vi "Retreive Target BuildSpecs.vi"(8 "error in (no error)":errorcluster, 10 "Target Names in":string[](array[string]), 11 "Project Sync Tools in":refnum<class "Project Sync Tools.lvclass">) -> (0 "error out":errorcluster, 2 "Target Names out":string[](array[string]), 3 "Project Sync Tools out":refnum<class "Project Sync Tools.lvclass">)   [LabVIEW 2019, in "Project Sync Tools.lvclass"]
uses:
  Project Sync Tools.lvclass
  TypeDefs/BuildSpec Parameters.ctl
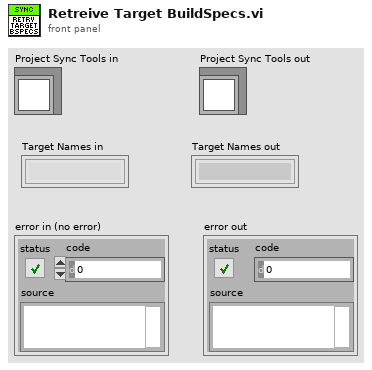
[diagram p1: front panel]
types:
  T1 = typedef "Project Sync Tools.lvclass/BuildSpec Parameters.ctl" = cluster{"BuildSpec Ref":refnum<vi>, "Target Name":string, "Build Spec Name":string, "Tags":string[], "Tag Values":variant[]}
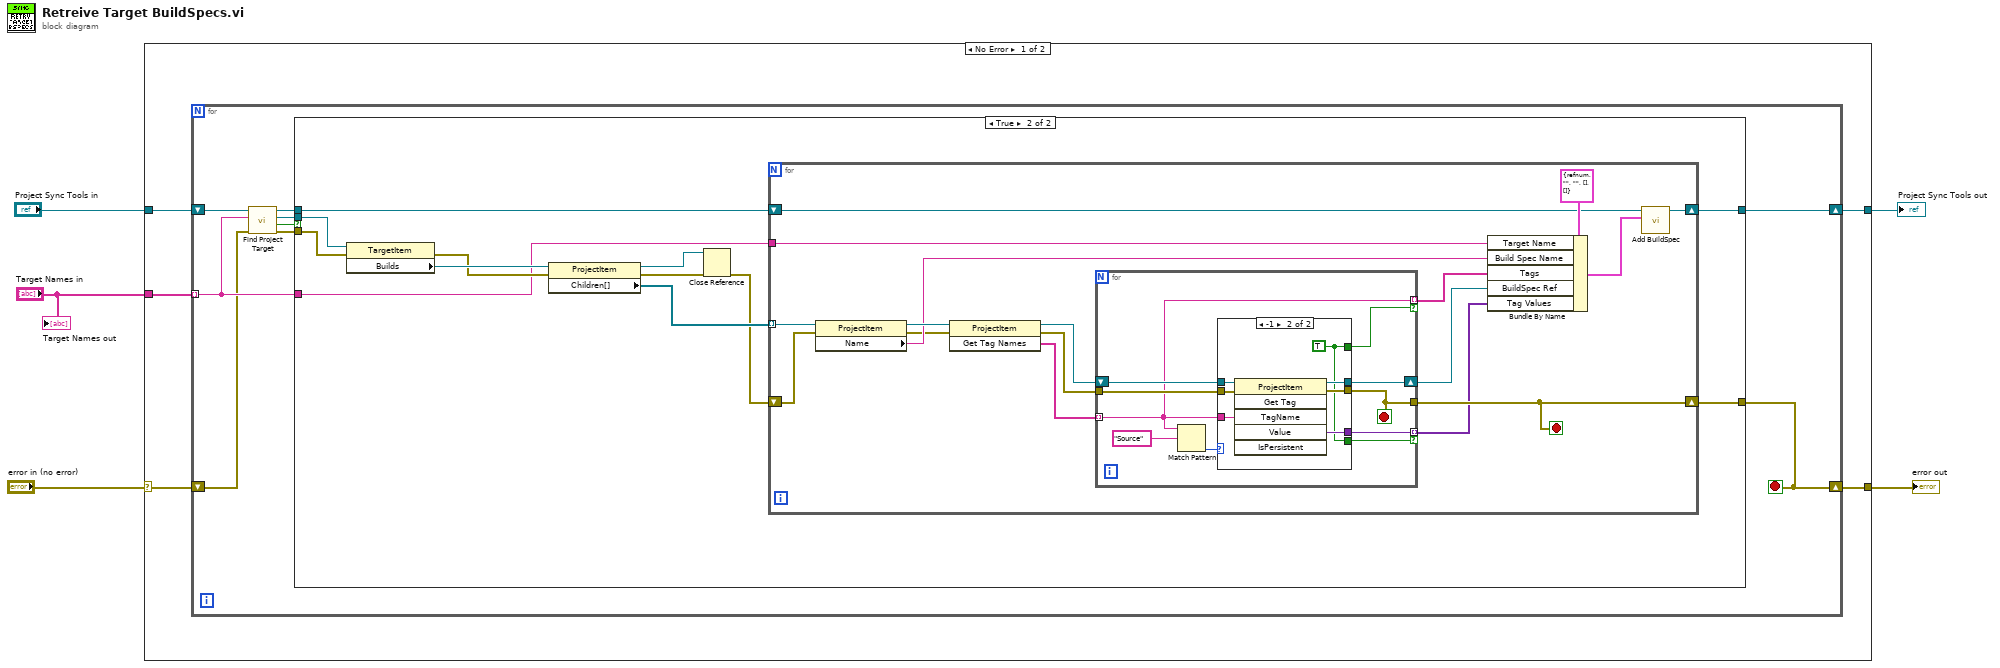
[diagram p0: block diagram]
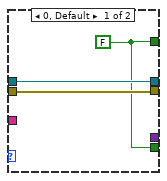
[diagram p3: hidden frame]
diagram:
  n1 = case shown="No Error" "error in (no error)" {
    selector: "error in (no error)" -> [w6 w72]
    tunnel: [w10 w71] -> w5
    tunnel: "Project Sync Tools in" -> [w9 w71]
    tunnel: "Target Names in" -> [w8 _]
    tunnel: [w7 w72] -> w3
    frame No Error {
      n2 = for {
        tunnel: w8 -> [w13] mode=indexing
        shift-right: [w19] -> w10
        shift-left: w9 -> [w17]
        shift-right: [w18] -> w7
        shift-left: w6 -> [w12]
        stop <- w18 stop-if-true
        n3 = call "Find Project Target.vi"("error in (no error)"=w12, "Target Name"=w13, "Project Sync Tools in"=w17) -> ("error out"=w11:errorcluster, "Found ?"=w16:bool, "TargetItem out"=w15:refnum<vi>, "Project Sync Tools out"=w14:refnum<class "Project Sync Tools.lvclass">)  [unwired: 5 in]
        n4 = case shown="True" w16 {
          tunnel: [w21 w31] -> w19
          tunnel: [w20 w27] -> w18
          tunnel: w15 -> [_ w25]
          tunnel: w14 -> [w21 w26]
          tunnel: w13 -> [_ w22]
          tunnel: w11 -> [w20 w24]
          frame False {
          }
          frame True {
            n5 = property class="TargetItem"(reference=w25, error in=w24) -> (error out=w23:errorcluster, "Builds"=w33:refnum<vi>)  [unwired: 1 out]
            n6 = property class="ProjectItem"(reference=w33, error in=w23) -> (reference out=w29:refnum<vi>, error out=w30:errorcluster, "Children[]"=w32:refnum<vi>[])
            n7 = Close Reference(reference=w29, error in (no error)=w30) -> (error out=w28:errorcluster)
            n8 = for {
              tunnel: w32 -> [w44] mode=indexing
              shift-right: [w45] -> w31
              shift-left: w26 -> [w46]
              tunnel: w22 -> [w42]
              shift-right: [w37] -> w27
              shift-left: w28 -> [w41]
              stop <- w37 stop-if-true
              n9 = property class="ProjectItem"(reference=w44, error in=w41) -> (reference out=w43:refnum<vi>, error out=w39:errorcluster, "Name"=w40:string)
              n10 = invoke class="ProjectItem" method="Get Tag Names"(reference=w43, error in=w39) -> (reference out=w50:refnum<vi>, error out=w38:errorcluster, "Get Tag Names"=w48:string[])  [unwired: 1 in]
              n11 = for {
                tunnel: w48 -> [w53] mode=indexing
                tunnel: [w59] -> w36 mode=indexing if=w52
                shift-right: [w58] -> w35
                shift-left: w50 -> [w60]
                tunnel: w38 -> [w57]
                tunnel: [w56] -> w37
                tunnel: [w53] -> w34 mode=indexing if=w51
                stop <- w56 stop-if-true
                n12 = Match Pattern(string=w53, regular expression="Source") -> (offset past match=w54:i32)  [unwired: 1 in, 3 out]
                n13 = case shown="-1" w54 {
                  tunnel: w60 -> [w63 w70]
                  tunnel: [_ w69] -> w59
                  tunnel: [w63 w68] -> w58
                  tunnel: w57 -> [w62 w67]
                  tunnel: [w62 w66] -> w56
                  tunnel: w53 -> [_ w65]
                  tunnel: [w61 w64] -> w52
                  tunnel: [w61 w64] -> w51
                  frame 0, Default {
                    w61 = FALSE
                  }
                  frame -1 {
                    w64 = TRUE
                    n14 = invoke class="ProjectItem" method="Get Tag"(reference=w70, error in=w67, "TagName"=w65) -> (reference out=w68:refnum<vi>, error out=w66:errorcluster, "Value"=w69:variant)  [unwired: 3 in, 3 out]
                  }
                }
              }
              n15 = Bundle By Name(cluster=T1 {"BuildSpec Ref"=refnum, "Target Name"="", "Build Spec Name"="", "Tags"=[], "Tag Values"=[]} ("Build Spec Parameters"), "Target Name"=w42, "Build Spec Name"=w40, "Tags"=w34, "BuildSpec Ref"=w35, "Tag Values"=w36) -> (w47:T1)
              n16 = call "Add BuildSpec.vi"("Build Spec Parameters"=w47, "Project Sync Tools in"=w46) -> ("Project Sync Tools out"=w45:refnum<class "Project Sync Tools.lvclass">)  [unwired: 8 in, 1 out]
            }
          }
        }
      }
    }
    frame Error {
    }
  }
  "Project Sync Tools out" <- w5
  "error out" <- w3
  "Target Names out" <- "Target Names in"
